vi "SetOutputMixerFrequency.vi"(8 "error in (no error)":errorcluster, 9 "Output enabled":bool=TRUE, 10 "Output mixer fequency [MHz]":dbl, 11 "FpgaRef5782 in":refnum<class "FpgaRef5782.lvclass">) -> (0 "error out":errorcluster, 3 "FpgaRef5782 out":refnum<class "FpgaRef5782.lvclass">)   [LabVIEW 2018, in "FpgaRef5782.lvclass"]
uses:
  FpgaRef5782.lvclass
  FpgaRef5782.lvclass/FpgaRef5782.ctl
  <vilib>/Utility/error.llb/Error Cluster From Error Code.vi
  <vilib>/rvi/errors/niLvFpgaAdjustHostInterfaceError.vi
  <vilib>/rvi/interface/nirviReadWriteControl/nirviReadWriteControl.xnode
  5782 FPGA ref.ctl
  NiFpgaLv.dll
  <vilib>/rvi/interface/Simulation/niFpgaSimulationCallBeginRW.vi
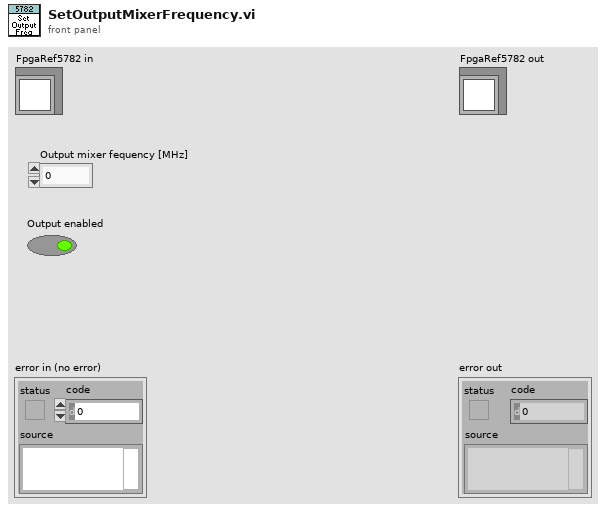
[diagram p1: front panel]
types:
  T1 = typedef "5782 FPGA ref.ctl" = refnum<k20>
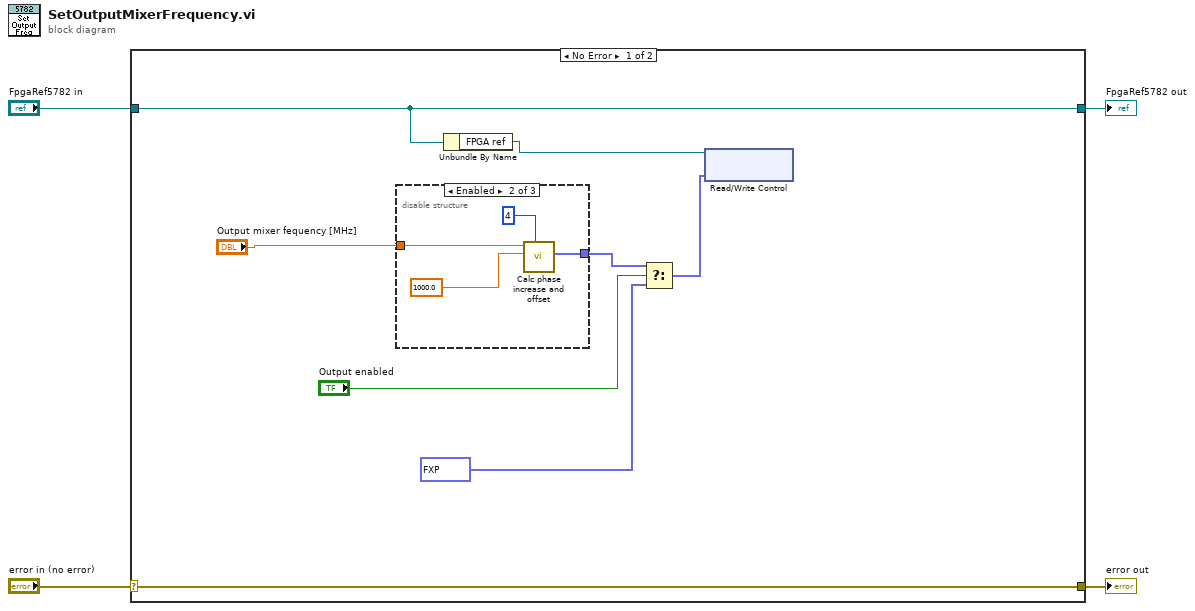
[diagram p0: block diagram]
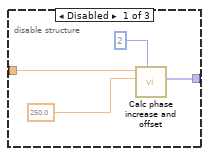
[diagram p2: hidden frame]
diagram:
  n1 = case shown="No Error" "error in (no error)" {
    selector: "error in (no error)" -> [w12 w22]
    tunnel: [w12 w22] -> w3
    tunnel: [w6 w21] -> w1
    tunnel: "FpgaRef5782 in" -> [w6 w21]
    frame No Error {
      n2 = disable-structure shown="Enabled" {
        disable-tunnel: [w14 w18 _] -> w8
        disable-tunnel: "Output mixer fequency [MHz]" -> [w13 w17 _]
        frame Disabled {
          n3 = call "Calc phase increase and offset.vi"("# of DDS"=2, "fclk (MHz)"=250.0 ("fclk (800MHz)"), "f_generated (MHz)"=w13) -> ("Phase out"=w14:fxp<+,64,64>[])  [unwired: 6 in, 2 out]
        }
        frame Enabled {
          n4 = call "Calc phase increase and offset.vi"("# of DDS"=4, "fclk (MHz)"=1000.0 ("fclk (800MHz)"), "f_generated (MHz)"=w17) -> ("Phase out"=w18:fxp<+,64,64>[])  [unwired: 6 in, 2 out]
        }
        frame Disabled {
        }
      }
      n5 = Unbundle By Name(w6) -> ("FPGA ref"=w5:T1)
      n6 = Select(t=w8, s="Output enabled", f=fxp<+,64,64>[] [0.0, 0.0, 0.0, 0.0, 0.0, 0.0, 0.0, 0.0, 0.0, 0.0, 0.0, 0.0, 0.0, 0.0, 0.0, 0.0]) -> (s? t:f=w7:fxp<+,64,64>[])
      n7 = xnode "Read/Write Control"("FPGA VI Reference In"=w5, "Phase output"=w7) -> ()  [unwired: 1 in, 2 out]
    }
    frame Error {
    }
  }
  "error out" <- w3
  "FpgaRef5782 out" <- w1
